vi "Set Fault Display Color.vi"(8 "error in (no error)":errorcluster, 11 "Fault Monitor in":refnum<class "Fault Monitor.lvclass">) -> (0 "error out":errorcluster, 3 "Fault Monitor out":refnum<class "Fault Monitor.lvclass">)   [LabVIEW 2023, in "Fault Monitor.lvlib" / "Fault Monitor.lvclass"]
uses:
  Library/Fault Monitor.lvclass
  Library/Fault Monitor.lvclass/Fault Monitor.ctl
  builds/Framework/Engine.lvlibp/Engine/Accessors/Read VI Ref.vi
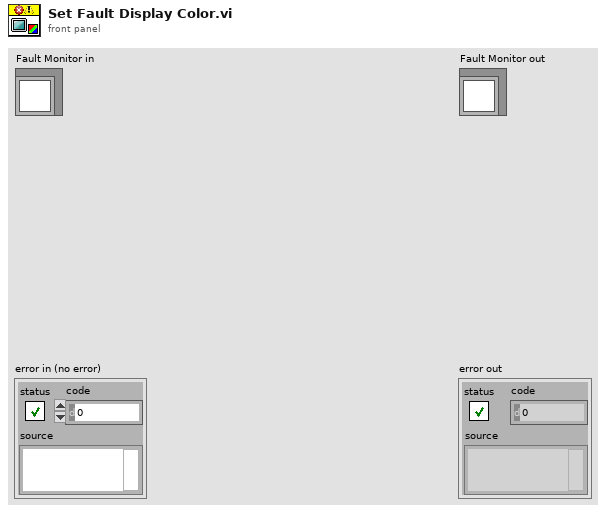
[diagram p1: front panel]
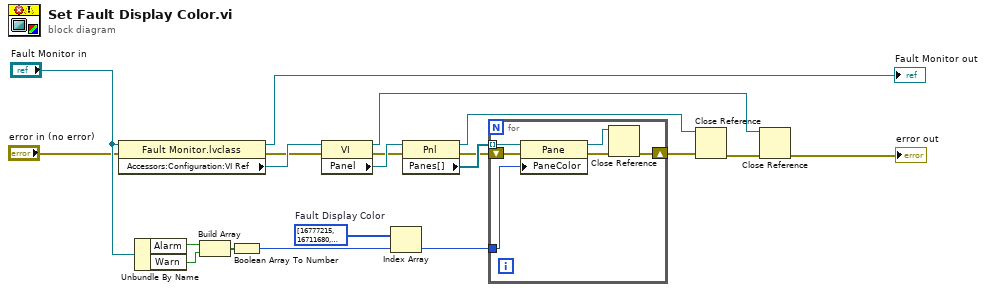
[diagram p0: block diagram]
diagram:
  w16 = u32[] [16777215, 16711680, 16383786, 16711680]  # Fault Display Color
  n1 = property class="Fault Monitor.lvclass"(reference="Fault Monitor in", error in="error in (no error)") -> (reference out=→"Fault Monitor out":refnum<class "Fault Monitor.lvclass">, error out=w11:errorcluster, "Accessors:Configuration:VI Ref"=w13:refnum<vi>)
  n2 = Unbundle By Name("Fault Monitor in") -> ("Alarm"=w20:bool, "Warn"=w19:bool)
  n3 = Build Array(w20, w19) -> (w18:bool[])
  n4 = Boolean Array To Number(Boolean array=w18) -> (number=w15:u32)
  n5 = property class="VI"(reference=w13, error in=w11) -> (reference out=w5:refnum<vi>, error out=w10:errorcluster, "Panel"=w14:refnum<vi>)
  n6 = Index Array(array=w16, index=w15) -> (element=w4:u32)
  n7 = property class="Pnl"(reference=w14, error in=w10) -> (reference out=w9:refnum<vi>, error out=w8:errorcluster, "Panes[]"=w12:refnum<vi>[])
  n8 = for {
    tunnel: w12 -> [w26] mode=indexing
    shift-right: [w24] -> w7
    shift-left: w8 -> [w25]
    tunnel: w4 -> [w21]
    n9 = property class="Pane"(reference=w26, error in=w25, "PaneColor"=w21) -> (reference out=w22:refnum<vi>, error out=w23:errorcluster)
    n10 = Close Reference(reference=w22, error in (no error)=w23) -> (error out=w24:errorcluster)
  }
  n11 = Close Reference(reference=w9, error in (no error)=w7) -> (error out=w6:errorcluster)
  n12 = Close Reference(reference=w5, error in (no error)=w6) -> (error out=→"error out":errorcluster)
